vi "Icon Editor Help.vi"   [LabVIEW 2021]
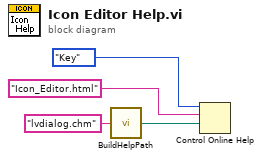
[diagram p0: block diagram]
diagram:
  n1 = call <vilib>:"BuildHelpPath.vi"("Help File Name"="lvdialog.chm") -> ("Help File Path"=w3:path)
  n2 = Control Online Help(2:w3, 3:"Icon_Editor.html" ("String to search for"), 4:enum16{"Contents", "Key", "Close"}."Key" ("Operation")) -> ()  [unwired: 1 in, 1 out]
